vi "READ Falcon500 values.vi"(0 "PhoenixMotorControlDevRef":T1, 1 "refnum name":string, 3 "error in (no error)":errorcluster) -> (6 "PhoenixMotorControlDevRef 2":T1={"DeviceStatus"={"status"=FALSE, "code"=0, "source"=""}, "Type"=enum."PWM", "PWM"={"PWM Channel"=enum."Invalid", "DeadBand"={"Name"="", "maxPositivePwm"=0, "minPositivePwm"=0, "centerPwm"=0, "maxNegativePwm"=0, "minNegativePwm"=0, "angularRange"=0}}, "CAN"={"Device Number"=0, "SetOutput VI Ref"=variant(enum8{"Percent VBus", "Current", "Speed", "Position", "Voltage"} enum."Percent VBus"), "GetOutput VI Ref"=variant(refnum<k1> refnum), "Enable VI Ref"=variant(dbl 12.0), "Disable VI Ref"=variant(enum8{"Percent VBus", "Speed", "Position", "Slave", "Unchanged / Invalid", "Voltage Compensation", "Current", "Motion Profile"} enum."Percent VBus"), "Data"=variant}, "Invert"=FALSE, "DIO PWM"={"PWM \"Enable\" Channel"=enum."Invalid", "DIOChannel"=enum."Invalid", "PWM Rate"=0.0}}, 9 "error out":errorcluster)   [LabVIEW 2020]
uses:
  <vilib>/Rock Robotics/WPI/MotorControl/WPI_MotorControlDeviceRef.ctl
  <vilib>/Rock Robotics/WPI/MotorControl/WPI_MotorControlType.ctl
  <vilib>/Rock Robotics/SystemInterfaces/DIO/FPGA_DIOPWMChannel.ctl
  <vilib>/Rock Robotics/WPI/PWM/WPI_PWMDeadband.ctl
  <vilib>/Rock Robotics/SystemInterfaces/DIO/FPGA_DIOChannel.ctl
  <vilib>/Rock Robotics/WPI/ThirdParty/Phoenix-LabVIEW/Motor Controller/Get/CTRE_Phoenix_MotorController_GetSelectedSensorData.vi
  <vilib>/Rock Robotics/Network Tables/NT Write Number.vi
  <vilib>/Rock Robotics/WPI/ThirdParty/Phoenix-LabVIEW/Motor Controller/Get/CTRE_Phoenix_MotorController_IntegratedSensorData_TalonFX.vi
  <vilib>/Rock Robotics/WPI/ThirdParty/Phoenix-LabVIEW/Motor Controller/Get/CTRE_Phoenix_MotorController_GetTemperature.vi
  <vilib>/Rock Robotics/WPI/ThirdParty/Phoenix-LabVIEW/Motor Controller/Get/CTRE_Phoenix_MotorController_GetLimitSwitchStates.vi
  <vilib>/Rock Robotics/Network Tables/NT Write Boolean.vi
panel:
  in  "ticks per rev":dbl=2048.0
  # "Note that the Falcon 500 encoder reports position as \"ticks\" of which there are 2048/rev and\nvelocity as ticks measured in a 100 ms period"
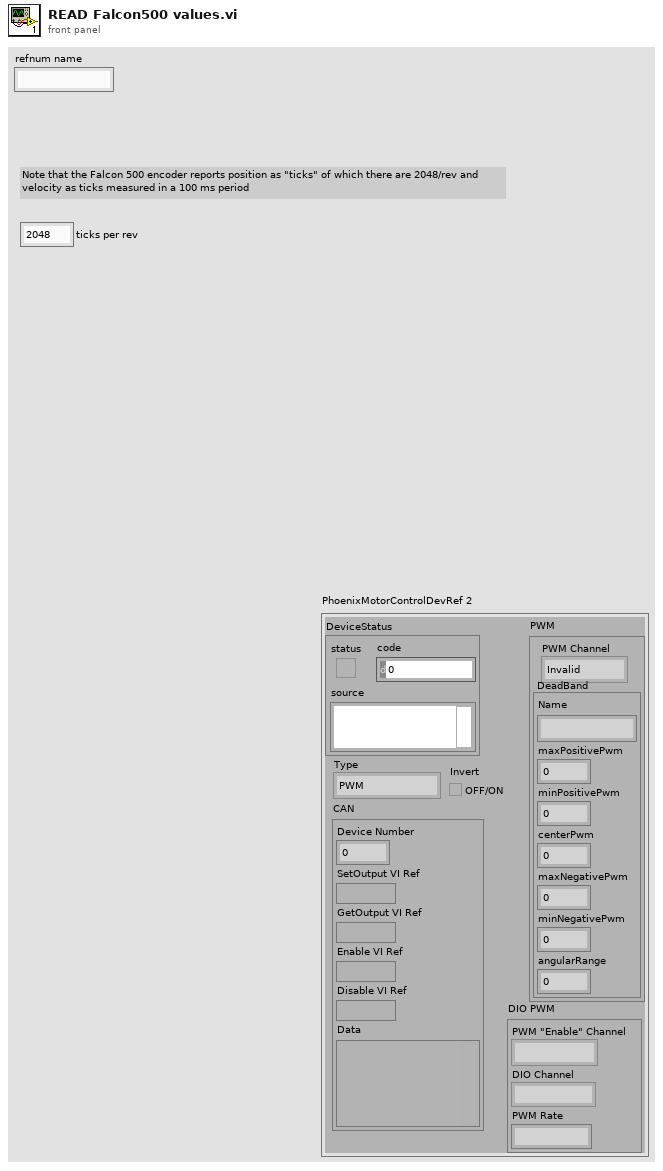
[diagram p1: front panel]
types:
  T1 = typedef "WPI_MotorControlDeviceRef.ctl" = cluster{"DeviceStatus":errorcluster, "Type":T2, "PWM":cluster{"PWM Channel":T3, "DeadBand":T4}, "CAN":cluster{"Device Number":u8, "SetOutput VI Ref":variant, "GetOutput VI Ref":variant, "Enable VI Ref":variant, "Disable VI Ref":variant, "Data":variant}, "Invert":bool, "DIO PWM":cluster{"PWM \"Enable\" Channel":T3, "DIOChannel":T5, "PWM Rate":dbl}}
  T2 = typedef "WPI_MotorControlType.ctl" = enum16{"PWM", "CAN", "DIO PWM"}
  T3 = typedef "FPGA_DIOPWMChannel.ctl" = enum8{"PWM 0", "PWM 1", "PWM 2", "PWM 3", "PWM 4", "PWM 5", "PWM 6", "PWM 7", "PWM 8", "PWM 9", "PWM MXP 0", "PWM MXP 1", "PWM MXP 2", "PWM MXP 3", "PWM MXP 4", "PWM MXP 5", "PWM MXP 6", "PWM MXP 7", "PWM MXP 8", "PWM MXP 9", "Invalid"}
  T4 = typedef "WPI_PWMDeadband.ctl" = cluster{"Name":string, "maxPositivePwm":i32, "minPositivePwm":i32, "centerPwm":i32, "maxNegativePwm":i32, "minNegativePwm":i32, "angularRange":u16}
  T5 = typedef "FPGA_DIOChannel.ctl" = enum8{"DIO 0", "DIO 1", "DIO 2", "DIO 3", "DIO 4", "DIO 5", "DIO 6", "DIO 7", "DIO 8", "DIO 9", "DIO MXP 0", "DIO MXP 1", "DIO MXP 2", "DIO MXP 3", "DIO MXP 4", "DIO MXP 5", "DIO MXP 6", "DIO MXP 7", "DIO MXP 8", "DIO MXP 9", "DIO MXP 10", "DIO MXP 11", "DIO MXP 12", "DIO MXP 13", "DIO MXP 14", "DIO MXP 15", "SPI Port CS1", "SPI Port CS2", "SPI Port CS3", "SPI Port MISO", "SPI Port MOSI", "Invalid"}
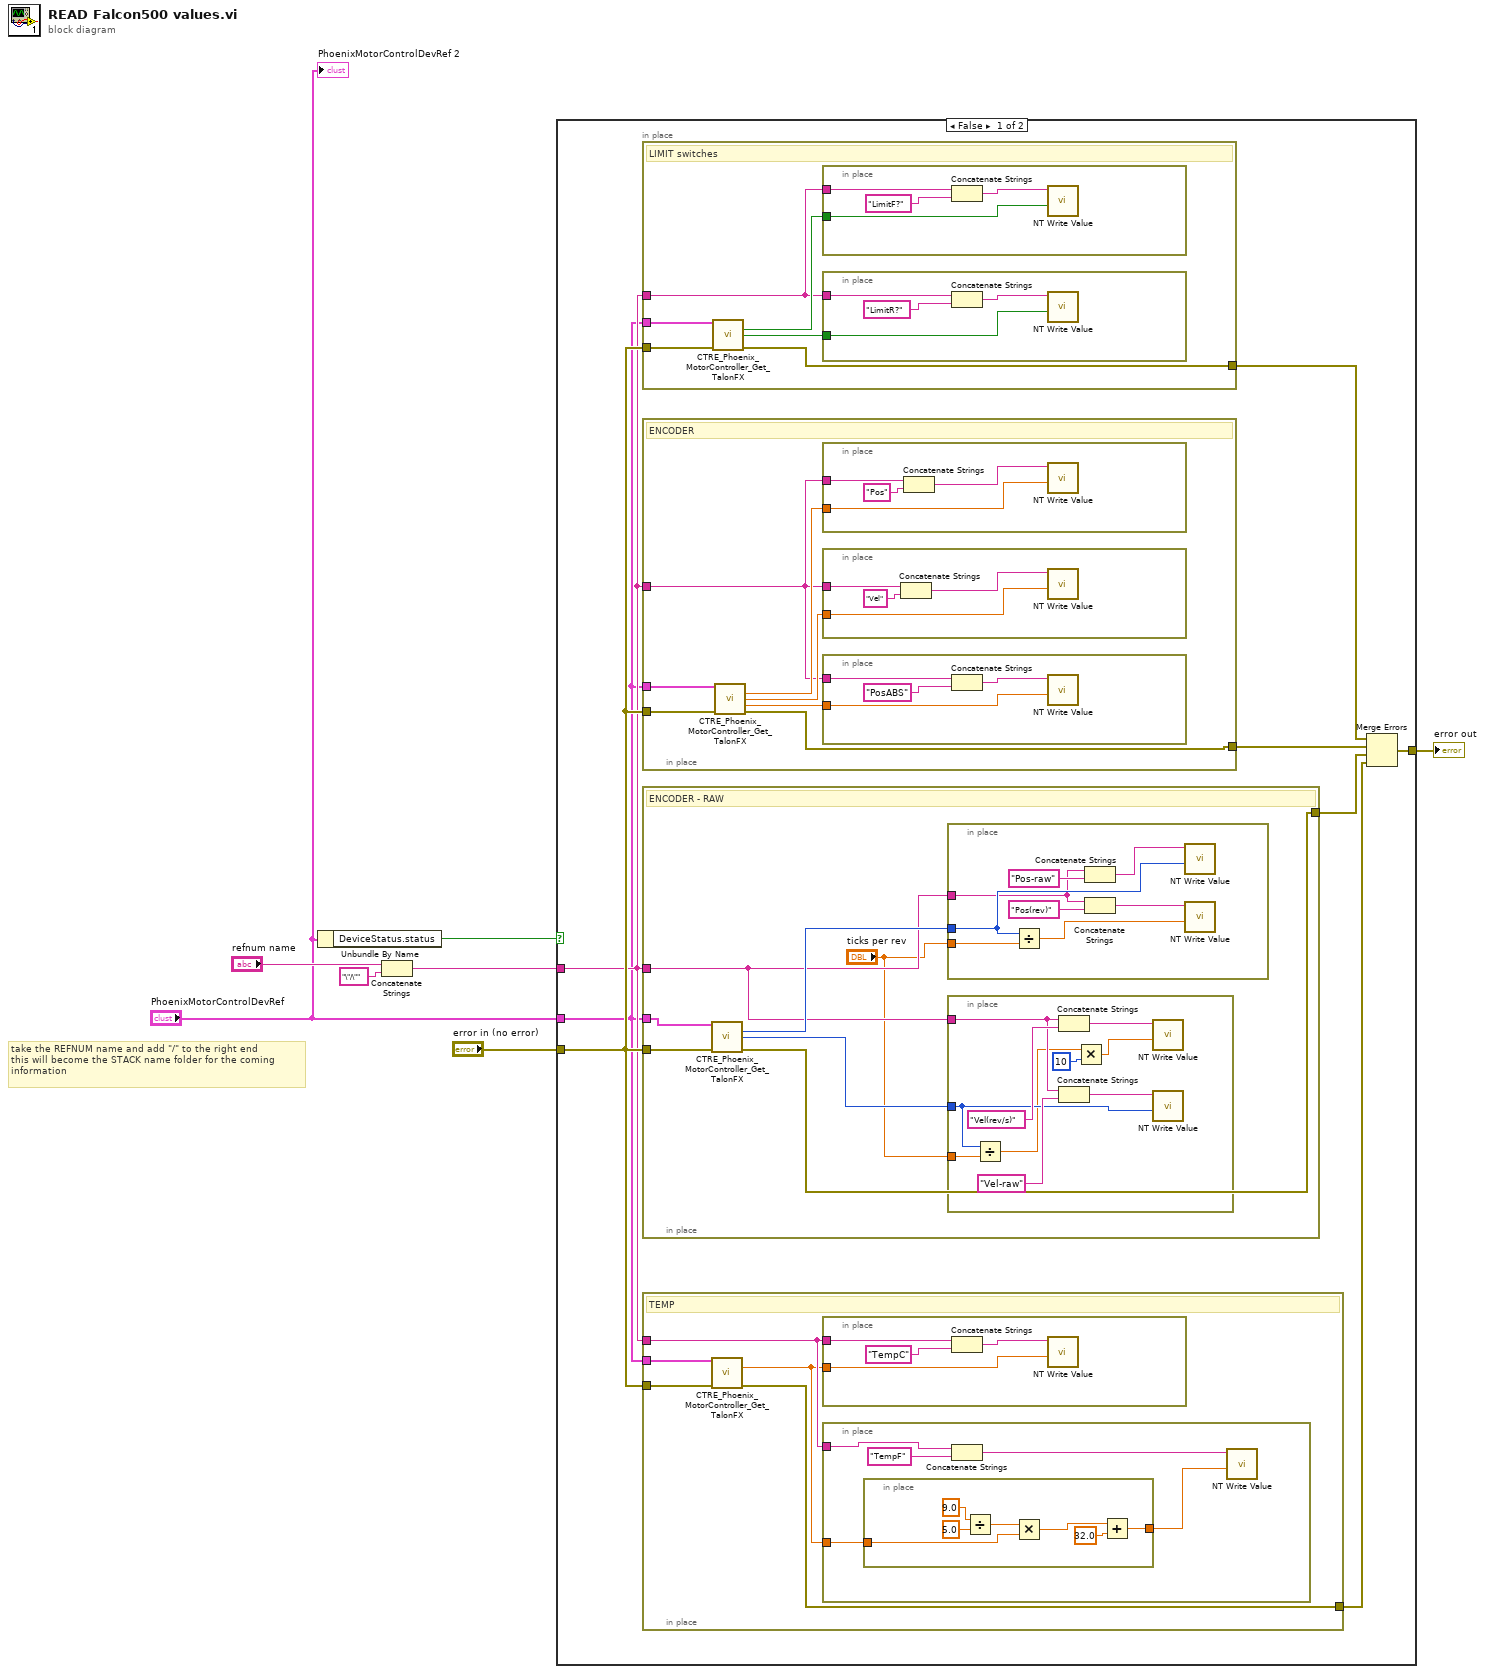
[diagram p0: block diagram]
diagram:
  # "take the REFNUM name and add \"/\" to the right end\nthis will become the STACK name folder for the coming\ninformation"
  n1 = Unbundle By Name("PhoenixMotorControlDevRef") -> ("DeviceStatus.status"=w2:bool)
  n2 = Concatenate Strings("refnum name", "\"/\"" ("string")) -> (w4:string)
  n3 = case shown="False" w2 {
    tunnel: "error in (no error)" -> [w15 _]
    tunnel: w4 -> [w14 _]
    tunnel: "PhoenixMotorControlDevRef" -> [w8 _]
    tunnel: [w13 _] -> w3
    frame False {
      n4 = in-place {
        in-place-border: w8 -> [w86]
        in-place-border: w15 -> [w85]
        in-place-border: [w82] -> w11
        in-place-border: w14 -> [w81]
        # "LIMIT switches"
        n5 = call-poly <vilib>:"CTRE_Phoenix_MotorController_Get_TalonFX.vi"("PhoenixMotorControlDevRef"=w86, "error in"=w85) -> ("Forward Limit Closed?"=w84:bool, "Reverse Limit Closed?"=w83:bool, "error out"=w82:errorcluster)  [unwired: 10 in, 1 out]
        n6 = in-place {
          in-place-border: w84 -> [w94]
          in-place-border: w81 -> [w93]
          n7 = Concatenate Strings(w93, "LimitF?" ("string")) -> (w92:string)
          n8 = call-poly <vilib>:"NT Write Value.vi"("Boolean"=w94, "Name"=w92) -> ()  [unwired: 9 in, 1 out]
        }
        n9 = in-place {
          in-place-border: w83 -> [w90]
          in-place-border: w81 -> [w89]
          n10 = Concatenate Strings(w89, "LimitR?" ("string")) -> (w88:string)
          n11 = call-poly <vilib>:"NT Write Value.vi"("Boolean"=w90, "Name"=w88) -> ()  [unwired: 9 in, 1 out]
        }
      }
      n12 = in-place {
        in-place-border: w8 -> [w68]
        in-place-border: [w64] -> w12
        in-place-border: w15 -> [w63]
        in-place-border: w14 -> [w62]
        # "ENCODER"
        n13 = call-poly <vilib>:"CTRE_Phoenix_MotorController_Get_TalonFX.vi"("PhoenixMotorControlDevRef"=w68, "error in"=w63) -> ("Position"=w67:dbl, "Velocity"=w66:dbl, "Absolute Position"=w65:dbl, "error out"=w64:errorcluster)  [unwired: 9 in, 1 out]
        n14 = in-place {
          in-place-border: w67 -> [w78]
          in-place-border: w62 -> [w77]
          n15 = Concatenate Strings(w77, "Pos" ("string")) -> (w80:string)
          n16 = call-poly <vilib>:"NT Write Value.vi"("Numeric"=w78, "Name"=w80) -> ()  [unwired: 9 in, 1 out]
        }
        n17 = in-place {
          in-place-border: w66 -> [w74]
          in-place-border: w62 -> [w73]
          n18 = Concatenate Strings(w73, "Vel" ("string")) -> (w76:string)
          n19 = call-poly <vilib>:"NT Write Value.vi"("Numeric"=w74, "Name"=w76) -> ()  [unwired: 9 in, 1 out]
        }
        n20 = in-place {
          in-place-border: w65 -> [w70]
          in-place-border: w62 -> [w69]
          n21 = Concatenate Strings(w69, "PosABS" ("string")) -> (w72:string)
          n22 = call-poly <vilib>:"NT Write Value.vi"("Numeric"=w70, "Name"=w72) -> ()  [unwired: 9 in, 1 out]
        }
      }
      n23 = in-place {
        in-place-border: w8 -> [w43]
        in-place-border: [w40] -> w10
        in-place-border: w15 -> [w39]
        in-place-border: w14 -> [w38]
        # "ENCODER - RAW"
        n24 = call-poly <vilib>:"CTRE_Phoenix_MotorController_Get_TalonFX.vi"("PhoenixMotorControlDevRef"=w43, "error in"=w39) -> ("Position (Raw Sensor Units)"=w42:i32, "Velocity (Raw Sensor Units per 100 ms)"=w41:i32, "error out"=w40:errorcluster)  [unwired: 10 in, 1 out]
        n25 = in-place {
          in-place-border: w42 -> [w59]
          in-place-border: w38 -> [w55]
          in-place-border: "ticks per rev" -> [w58]
          n26 = Divide(x=w59, y=w58) -> (x/y=w54:dbl)
          n27 = Concatenate Strings(w55, "Pos-raw" ("string")) -> (w61:string)
          n28 = Concatenate Strings(w55, "Pos(rev)" ("string")) -> (w56:string)
          n29 = call-poly <vilib>:"NT Write Value.vi"("Numeric"=w59, "Name"=w61) -> ()  [unwired: 9 in, 1 out]
          n30 = call-poly <vilib>:"NT Write Value.vi"("Numeric"=w54, "Name"=w56) -> ()  [unwired: 9 in, 1 out]
        }
        n31 = in-place {
          in-place-border: w41 -> [w46]
          in-place-border: w38 -> [w49]
          in-place-border: "ticks per rev" -> [w47]
          n32 = Divide(x=w46, y=w47) -> (x/y=w45:dbl)
          n33 = Concatenate Strings(w49, "Vel(rev/s)" ("string")) -> (w51:string)
          n34 = Concatenate Strings(w49, "Vel-raw" ("string")) -> (w53:string)
          n35 = Multiply(x=w45, y=10) -> (x*y=w44:dbl)
          n36 = call-poly <vilib>:"NT Write Value.vi"("Numeric"=w44, "Name"=w51) -> ()  [unwired: 9 in, 1 out]
          n37 = call-poly <vilib>:"NT Write Value.vi"("Numeric"=w46, "Name"=w53) -> ()  [unwired: 9 in, 1 out]
        }
      }
      n38 = in-place {
        in-place-border: w8 -> [w20]
        in-place-border: [w19] -> w9
        in-place-border: w15 -> [w18]
        in-place-border: w14 -> [w17]
        # "TEMP"
        n39 = call-poly <vilib>:"CTRE_Phoenix_MotorController_Get_TalonFX.vi"("PhoenixMotorControlDevRef"=w20, "error in"=w18) -> ("Temperature (C)"=w16:dbl, "error out"=w19:errorcluster)  [unwired: 11 in, 1 out]
        n40 = in-place {
          in-place-border: w16 -> [w34]
          in-place-border: w17 -> [w33]
          n41 = Concatenate Strings(w33, "TempC" ("string")) -> (w36:string)
          n42 = call-poly <vilib>:"NT Write Value.vi"("Numeric"=w34, "Name"=w36) -> ()  [unwired: 9 in, 1 out]
        }
        n43 = in-place {
          in-place-border: w17 -> [w23]
          in-place-border: w16 -> [w22]
          n44 = in-place {
            in-place-border: w22 -> [w32]
            in-place-border: [w29] -> w21
            n45 = Divide(x=9.0, y=5.0) -> (x/y=w27:dbl)
            n46 = Multiply(x=w27, y=w32) -> (x*y=w30:dbl)
            n47 = Add(x=w30, y=32.0) -> (x+y=w29:dbl)
          }
          n48 = Concatenate Strings(w23, "TempF" ("string")) -> (w25:string)
          n49 = call-poly <vilib>:"NT Write Value.vi"("Numeric"=w21, "Name"=w25) -> ()  [unwired: 9 in, 1 out]
        }
      }
      n50 = Merge Errors(w11, w12, w10, w9) -> (w13:errorcluster)
    }
    frame True {
    }
  }
  "error out" <- w3
  "PhoenixMotorControlDevRef 2" <- "PhoenixMotorControlDevRef"
